vi "Guid Generator.vi"(8 "error in (no error)":errorcluster) -> (0 "error out":errorcluster, 2 "GUID":string)   [LabVIEW 2016]
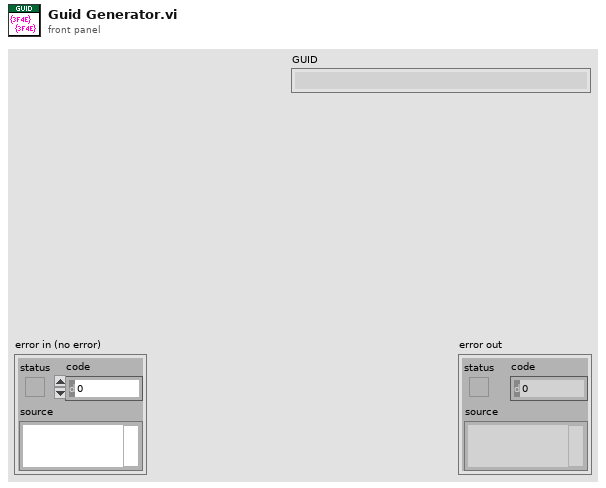
[diagram p1: front panel]
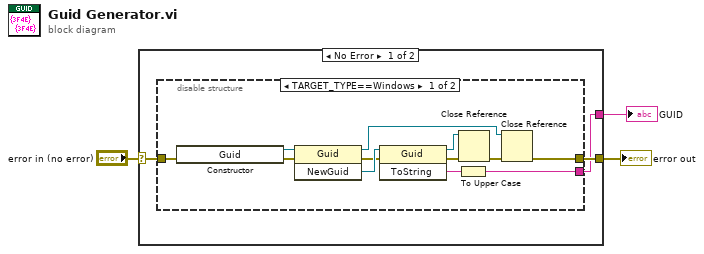
[diagram p0: block diagram]
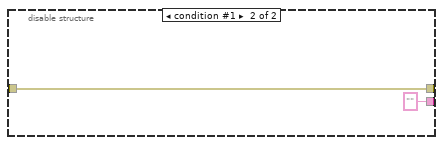
[diagram p2: hidden frame]
diagram:
  n1 = case shown="No Error" "error in (no error)" {
    selector: "error in (no error)" -> [w6 _]
    tunnel: [w5 _] -> w2
    tunnel: [w4 _] -> w1
    frame No Error {
      n2 = disable-structure shown="TARGET_TYPE==Windows" {
        disable-tunnel: w6 -> [w9 w20]
        disable-tunnel: [w8 w20] -> w5
        disable-tunnel: [w7 ""] -> w4
        frame condition #0 (active) {
          n3 = constructor class="System.Guid" ("Constructor Node")(error in=w9) -> (reference out=w18:refnum<k24>, error out=w17:errorcluster)  [unwired: 2 in, 1 out]
          n4 = invoke class="Guid" method="NewGuid"(reference=w18, error in=w17) -> (reference out=w12:refnum<k24>, error out=w15:errorcluster, "NewGuid"=w16:refnum<k24>)  [unwired: 1 in]
          n5 = invoke class="Guid" method="ToString"(reference=w16, error in=w15) -> (reference out=w13:refnum<k24>, error out=w14:errorcluster, "ToString"=w10:string)  [unwired: 1 in]
          n6 = To Upper Case(1:w10) -> (0:w7:string)
          n7 = Close Reference(reference=w13, error in (no error)=w14) -> (error out=w11:errorcluster)
          n8 = Close Reference(reference=w12, error in (no error)=w11) -> (error out=w8:errorcluster)
        }
        frame condition #1 {
        }
      }
    }
    frame Error {
    }
  }
  "error out" <- w2
  "GUID" <- w1
